vi "Caterpillar Error Handler.vi"(7 "Error State":string, 8 "Back Leg Up":bool, 9 "Mid Leg Up":bool, 10 "Front Leg Up":bool, 11 "state in":string) -> (1 "Error Text":string, 3 "state out":string)   [LabVIEW 2012]
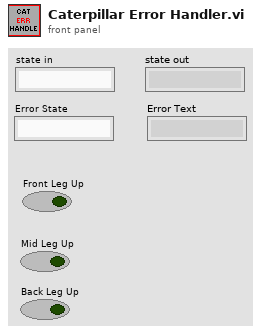
[diagram p1: front panel]
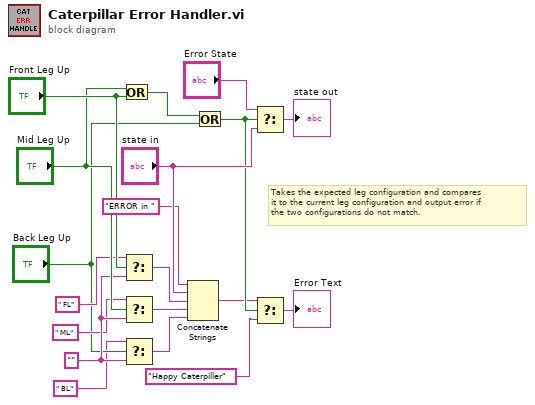
[diagram p0: block diagram]
diagram:
  w9 = "" ("f")
  # "Takes the expected leg configuration and compares\nit to the current leg configuration and output error if \nthe two configurations do not match."
  n1 = Or(x="Mid Leg Up", y="Front Leg Up") -> (x .or. y?=w18:bool)
  n2 = Select(t=" FL" ("f"), s="Front Leg Up", f=w9) -> (s? t:f=w4:string)
  n3 = Select(t=" ML" ("f"), s="Mid Leg Up", f=w9) -> (s? t:f=w3:string)
  n4 = Select(t=" BL" ("f"), s="Back Leg Up", f=w9) -> (s? t:f=w2:string)
  n5 = Concatenate Strings("ERROR in " ("string"), "state in", w4, w3, w2) -> (w13:string)
  n6 = Or(x=w18, y="Back Leg Up") -> (x .or. y?=w14:bool)
  n7 = Select(t="Error State", s=w14, f="state in") -> (s? t:f=→"state out":string)
  n8 = Select(t=w13, s=w14, f="Happy Caterpiller") -> (s? t:f=→"Error Text":string)
